vi "OP300ZP_prep bdd init.vi"(10 "tabin":string[](array[string]), 11 "type":i32) -> (3 "Tableau":string[](array[string]))   [LabVIEW 2020]
uses:
  OP300ZP_selectdata.ctl
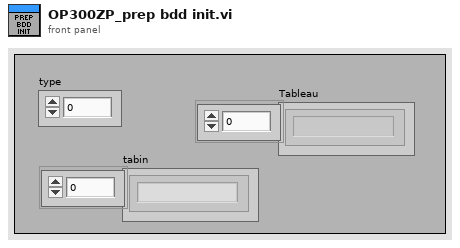
[diagram p1: front panel]
types:
  T1 = typedef "OP300ZP_selectdata.ctl" = u16
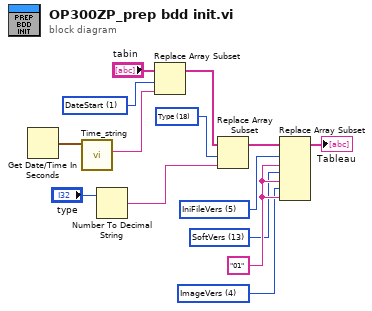
[diagram p0: block diagram]
diagram:
  w6 = T1 4 items=["IdOp300", "DateStart", "DeltaTC", "DeltaVC", "ImageVers", "IniFileVers", "InsuN", "InsuP", "MCU", "OCV", "Operateur", "Pass", "SN", "SoftVers", "TC0", "TC1", "TempsTest", "Tfactory", "Type", "VC0", "VC1"] ("Menu déroulant")
  w4 = T1 13 items=["IdOp300", "DateStart", "DeltaTC", "DeltaVC", "ImageVers", "IniFileVers", "InsuN", "InsuP", "MCU", "OCV", "Operateur", "Pass", "SN", "SoftVers", "TC0", "TC1", "TempsTest", "Tfactory", "Type", "VC0", "VC1"] ("Menu déroulant")
  w5 = T1 5 items=["IdOp300", "DateStart", "DeltaTC", "DeltaVC", "ImageVers", "IniFileVers", "InsuN", "InsuP", "MCU", "OCV", "Operateur", "Pass", "SN", "SoftVers", "TC0", "TC1", "TempsTest", "Tfactory", "Type", "VC0", "VC1"] ("Menu déroulant")
  w7 = T1 18 items=["IdOp300", "DateStart", "DeltaTC", "DeltaVC", "ImageVers", "IniFileVers", "InsuN", "InsuP", "MCU", "OCV", "Operateur", "Pass", "SN", "SoftVers", "TC0", "TC1", "TempsTest", "Tfactory", "Type", "VC0", "VC1"] ("Menu déroulant")
  w8 = T1 1 items=["IdOp300", "DateStart", "DeltaTC", "DeltaVC", "ImageVers", "IniFileVers", "InsuN", "InsuP", "MCU", "OCV", "Operateur", "Pass", "SN", "SoftVers", "TC0", "TC1", "TempsTest", "Tfactory", "Type", "VC0", "VC1"] ("Menu déroulant")
  w12 = "01" ("nouvel élément/sous-tableau")
  n1 = Get Date/Time In Seconds() -> (seconds since 1Jan1904=w14:timestamp)
  n2 = call <userlib>:"Time_string.vi"("h in"=w14) -> ("heure sql"=w13:string)  [unwired: 9 in, 1 out]
  n3 = Number To Decimal String(number="type") -> (decimal integer string=w3:string)  [unwired: 1 in]
  n4 = Replace Array Subset(array="tabin", new element=w13, index=w8) -> (w11:string[])
  n5 = Replace Array Subset(array=w11, new element=w3, index=w7) -> (w9:string[])
  n6 = Replace Array Subset(array=w9, new element #1=w12, index #1=w5, new element #2=w12, index #2=w4, new element #3=w12, index #3=w6) -> (→"Tableau":string[])
